vi "touch and led.vi"() -> ()   [LabVIEW 2019]
panel:
  in  "stop (F)":bool
  out "touch":dbl
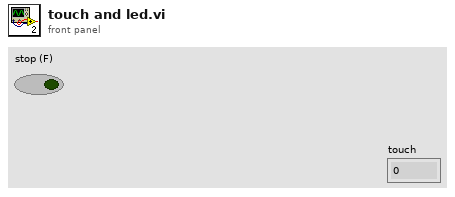
[diagram p1: front panel]
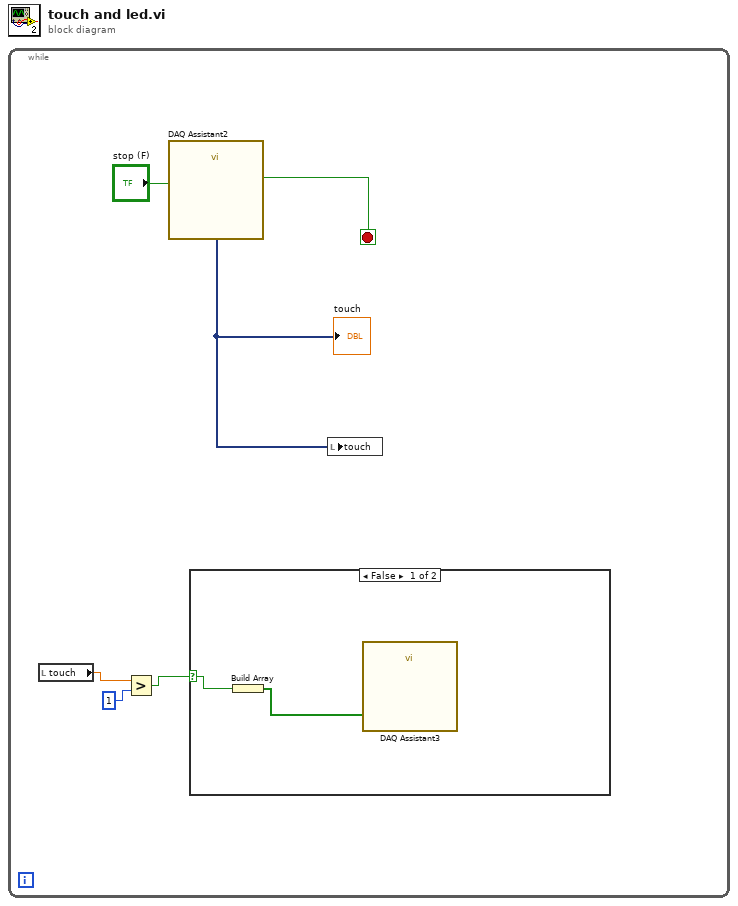
[diagram p0: block diagram]
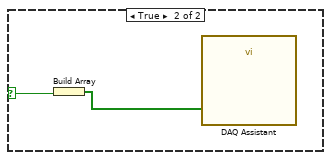
[diagram p2: hidden frame]
diagram:
  n1 = while {
    stop <- w5 stop-if-true
    n2 = local read "touch"() -> (w3:dbl)
    n3 = Greater?(x=w3, y=1) -> (0:w1:bool)
    n4 = call "DAQ Assistant2"("stop (F)"="stop (F)") -> ("data"=w4:dynamicdata, "stopped"=w5:bool)  [unwired: 15 in, 2 out]
    "touch" <- w4
    n5 = case shown="False" w1 {
      selector: w1 -> [w8 w10]
      frame False {
        n6 = Build Array(w8) -> (w7:bool[])
        n7 = call "DAQ Assistant3"("data"=w7) -> ()  [unwired: 17 in, 2 out]
      }
      frame True {
        n8 = Build Array(w10) -> (w9:bool[])
        n9 = call "DAQ Assistant"("data"=w9) -> ()  [unwired: 17 in, 2 out]
      }
    }
    n10 = local write "touch"(w4) -> ()
  }
